vi "FilterEvent0.vi"() -> ()   [LabVIEW 2020]
panel:
  in  "Stop":bool
  in  "Control":u16
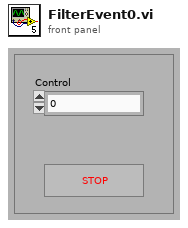
[diagram p1: front panel]
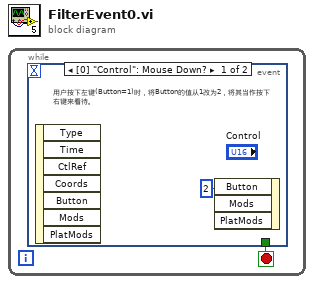
[diagram p0: block diagram]
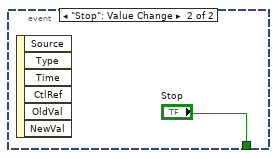
[diagram p2: hidden frame]
diagram:
  n1 = while {
    stop <- w1 stop-if-true
    n2 = event shown="[0] \"Control\": Mouse Down?" {
      selector: _ -> [_ _]
      dyn-events: _ -> [_ _]
      timeout: _ -> [_ _]
      tunnel: [_ "Stop"] -> w1
      event "Control": Mouse Down? {
        # "用户按下左键(Button=1)时，将Button的值从1改为2，将其当作按下右键来看待。"
        n3 = event-data() -> ()  [unwired: 8 out]
        n4 = event-data("Button"=u16 2) -> ()  [unwired: 1 in, 3 out]
      }
      event "Stop": Value Change {
        n5 = event-data() -> ()  [unwired: 7 out]
      }
    }
  }
